vi "RT Driver VI.vi"(7 "Operation":T1, 11 "Device Reference in":T2 format="%.0x") -> (0 "Error Code":i32)   [LabVIEW 2015, in "Diagnostics Addon Engine.lvlib"]
uses:
  Diagnostics Addon Engine.lvlib
  <vilib>/NI Veristand/Custom Device API/Custom Device Item Ref.ctl
  <vilib>/NI Veristand/Custom Device API/Hardware Interface Driver VI Operation.ctl
  SubVIs/Inline Async API/Controls/Parameters Cluster.ctl
  SubVIs/Error Handling API/Controls/Error Handling Cluster.ctl
  SubVIs/VS Data Channels.ctl
  SubVIs/Inline Async API/Controls/Write To VS Engine.ctl
  <vilib>/NI Veristand/Custom Device API/Data Reference.ctl
  SubVIs/Inline Async API/Controls/Read From VS Engine.ctl
  <vilib>/NI Veristand/Custom Device API/Block Data Reference.ctl
  SubVIs/Inline Async API/Controls/ReadWrite Data.ctl
  SubVIs/Compiled.Settings
  SubVIs/Section Properties.ctl
  Shared/CAN Configuration.ctl
  Shared/CAN Interface.ctl
  Shared/Diagnostic Protocols.ctl
  Shared/Transport Protocols.ctl
  Shared/Security.ctl
  Shared/FPGA Bitfile Settings.ctl
  Shared/Frame Parameters.ctl
  Shared/Signal Parameters.ctl
  Shared/DPID Parameters.ctl
  Shared/DPID Periodic Rate.ctl
  <vilib>/Automotive Diagnostic Command Set/Diagnostic Protocols.llb/DTC Descriptor.ctl
  Shared/Compiled.Refs.ctl
  SubVIs/Inline Async API/Initialize Read From VS Engine.vi
  <vilib>/NI Veristand/Custom Device API/NI VeriStand - Set Channel Value by Data Reference.vi
  <vilib>/NI Veristand/Custom Device API/NI VeriStand - Get Channel Value by Data Reference.vi
  <vilib>/NI Veristand/Custom Device API/NI VeriStand - Get Channel Values by Block Data Reference.vi
  SubVIs/Error Handling API/Print/Display and Log Custom Device Error.vi
  Shared/GUID Lookup.vi
  <vilib>/NI Veristand/Custom Device API/Get Item Property (Variant).vi
  SubVIs/Read and Load Bitfile.vi
  SubVIs/Inline Async API/Initialize ReadWrite Data.vi
  SubVIs/Inline Async API/Initialize Write Data to VS Engine.vi
  <vilib>/NI Veristand/Custom Device API/Global Data Refs.vi
  SubVIs/Inline Async API/Inline Async API.lvlib
  SubVIs/Error Handling API/Error Handling API.lvlib
  <vilib>/NI Veristand/Custom Device API/Custom Device API.lvlib
  <vilib>/NI Veristand/Custom Device Tools/Custom Device Utility Library/Custom Device Utility Library.lvlib
  Shared/Diagnostics Addon Shared.lvlib
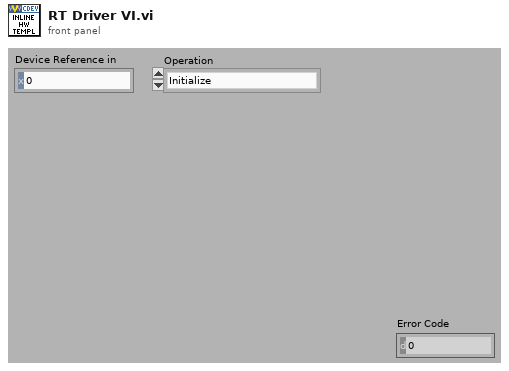
[diagram p1: front panel]
types:
  T1 = typedef "Custom Device API.lvlib/Hardware Interface Driver VI Operation.ctl" = enum16{"Initialize", "Start", "Read Data from HW", "Write Data to HW", "Close"}
  T2 = typedef "Custom Device API.lvlib/Custom Device Item Ref.ctl" = u64
  T3 = typedef "Diagnostics Addon Engine.lvlib/Error Handling API.lvlib/Error Handling Cluster.ctl" = cluster{"Error Process Q":refnum<queue>, "Process Qs":refnum<queue>[]}
  T4 = typedef "Diagnostics Addon Engine.lvlib/VS Data Channels.ctl" = cluster{"ToVS.PIDs":T5, "ToVS.DIDs":T5, "ToVS.DTCs":T5, "ToVS.DTCCount":T5, "ToVS.Success":T5, "FromVS.CPIDs":T7, "Cmds":T9}
  T5 = typedef "Diagnostics Addon Engine.lvlib/Inline Async API.lvlib/Write To VS Engine.ctl" = cluster{"Name":string, "Write to VS Engine FIFO":refnum<k33>, "Pairs":cluster{"Refs":T6[], "Values":dbl[]}}
  T6 = typedef "Custom Device API.lvlib/Data Reference.ctl" = i32
  T7 = typedef "Diagnostics Addon Engine.lvlib/Inline Async API.lvlib/Read From VS Engine.ctl" = cluster{"Name":string, "Read from VS Engine FIFO":refnum<k33>, "Pairs":cluster{"Refs":T8[], "Values":dbl[]}}
  T8 = typedef "Custom Device API.lvlib/Block Data Reference.ctl" = cluster{"Data Reference":T6, "Offset":u64, "Length":u64}
  T9 = typedef "Diagnostics Addon Engine.lvlib/Inline Async API.lvlib/ReadWrite Data.ctl" = cluster{"Name":string, "Write to VS Engine FIFO":refnum<k33>, "Read from VS Engine FIFO":refnum<k33>, "Pairs":cluster{"Chan Refs":T6[], "Prev. Values":dbl[]}}
  T10 = cluster{"Device Error":errorcluster, "VI Refs":refnum<vi>[], "Error Handling Cluster":T3, "ChanRefs":T4, "FPGA Session":u32}
  T11 = typedef "Diagnostics Addon Shared.lvlib/Compiled.Settings" = cluster{"Properties":T12, "Refs":T24}
  T12 = typedef "Diagnostics Addon Engine.lvlib/Section Properties.ctl" = cluster{"Name":string, "CAN":T13, "FPGA Settings":T18, "PIDs":T19[], "PID Lookup":variant, "CPIDs":T19[], "CPID Lookup":variant, "DIDs":T19[], "DID Lookup":variant, "DPIDs":T21[], "DPID Lookup":variant, "DTC descriptor":T23}
  T13 = typedef "Diagnostics Addon Shared.lvlib/CAN Configuration.ctl" = cluster{"Database File":path, "CAN Interface":T14, "Baud Rate":u32, "Diagnostic Protocol":T15, "Transport Protocol":T16, "Transmit ID":u32, "Receive ID":u32, "Transmit Extension":u8, "Receive Extension":u8, "Receive UUDT ID":u32, "Enable Stream":bool, "VW TP Channel ID":u32, "Security":T17}
  T14 = typedef "Diagnostics Addon Shared.lvlib/CAN Interface.ctl" = enum16{"CAN0", "CAN1", "CAN2", "CAN3", "CAN4", "CAN5", "CAN6", "CAN7", "CAN8", "CAN9", "CAN10", "CAN11", "CAN12", "CAN13", "CAN14", "CAN15", "CAN16", "CAN17", "CAN18", "CAN19", "CAN20", "CAN21", "CAN22", "CAN23", "CAN24", "CAN25", "CAN26", "CAN27", "CAN28", "CAN29", "CAN30", "CAN31", "CAN32", "CAN33", "CAN34", "CAN35", "CAN36", "CAN37", "CAN38", "CAN39", "CAN40", "CAN41", "CAN42", "CAN43", "CAN44", "CAN45", "CAN46", "CAN47", "CAN48", "CAN49", "CAN50", "CAN51", "CAN52", "CAN53", "CAN54", "CAN55", "CAN56", "CAN57", "CAN58", "CAN59", "CAN60", "CAN61", "CAN62", "CAN63", "CAN 256 (Virtual)", "CAN 257 (Virtual)"}
  T15 = typedef "Diagnostics Addon Shared.lvlib/Diagnostic Protocols.ctl" = enum16{"GMLAN", "KWP-2000", "UDS"}
  T16 = typedef "Diagnostics Addon Shared.lvlib/Transport Protocols.ctl" = enum16{"ISO TP - Normal Mode", "ISO TP - Mixed Mode", "VW TP 2.0", "Diagnostics on IP"}
  T17 = typedef "Diagnostics Addon Shared.lvlib/Security.ctl" = cluster{"DLL Path":path, "Security Level":u8}
  T18 = typedef "Diagnostics Addon Shared.lvlib/FPGA Bitfile Settings.ctl" = cluster{"RT Bitfile Path":path, "RIO Device":u16, "Enable":bool}
  T19 = typedef "Diagnostics Addon Shared.lvlib/Frame Parameters.ctl" = cluster{"Name":string, "Description":string, "ID":u16, "Signals":T20[]}
  T20 = typedef "Diagnostics Addon Shared.lvlib/Signal Parameters.ctl" = cluster{"Start Bit":u8, "Length":u8, "Scaling Factor":dbl, "Scaling Offset":dbl, "Minimum":dbl, "Maximum":dbl, "Data Type":u32, "Byte Order":u32, "Default Value":dbl, "Name":string, "Units":string, "Description":string}
  T21 = typedef "Diagnostics Addon Shared.lvlib/DPID Parameters.ctl" = cluster{"DPID ID":u8, "Speed":T22, "PIDs":u16[]}
  T22 = typedef "Diagnostics Addon Shared.lvlib/DPID Periodic Rate.ctl" = enum16{"Slow", "Medium", "Fast"}
  T23 = typedef "Diagnostics Addon Shared.lvlib/DTC Descriptor.ctl" = cluster{"DTC Byte Length":i32, "Status Byte Length":i32, "Add Data Byte Length":i32, "Byte Order":enum16{"Motorola", "Intel"}}
  T24 = typedef "Diagnostics Addon Shared.lvlib/Compiled.Refs.ctl" = cluster{"PIDs":T6[], "CPIDs":cluster{"Refs":T8[], "Values":dbl[]}, "DIDs":T6[], "Number of DTCs":T6, "DTCs":T6[], "Success":T6, "Command Chanels":T6[]}
  T25 = typedef "Diagnostics Addon Engine.lvlib/Inline Async API.lvlib/Parameters Cluster.ctl" = cluster{"Parameter Name":string, "Initial Settings":variant}
  T26 = typedef "Diagnostics Addon Engine.lvlib/Main Configuration.ctl" = cluster{"Properties":T12, "ChanRefs":T4}
  T27 = cluster{"Chan Refs":T6[], "Previous Chan Values":dbl[]}
  T28 = cluster{"Block Data Refs":T8[], "Previous Chan Values":dbl[]}
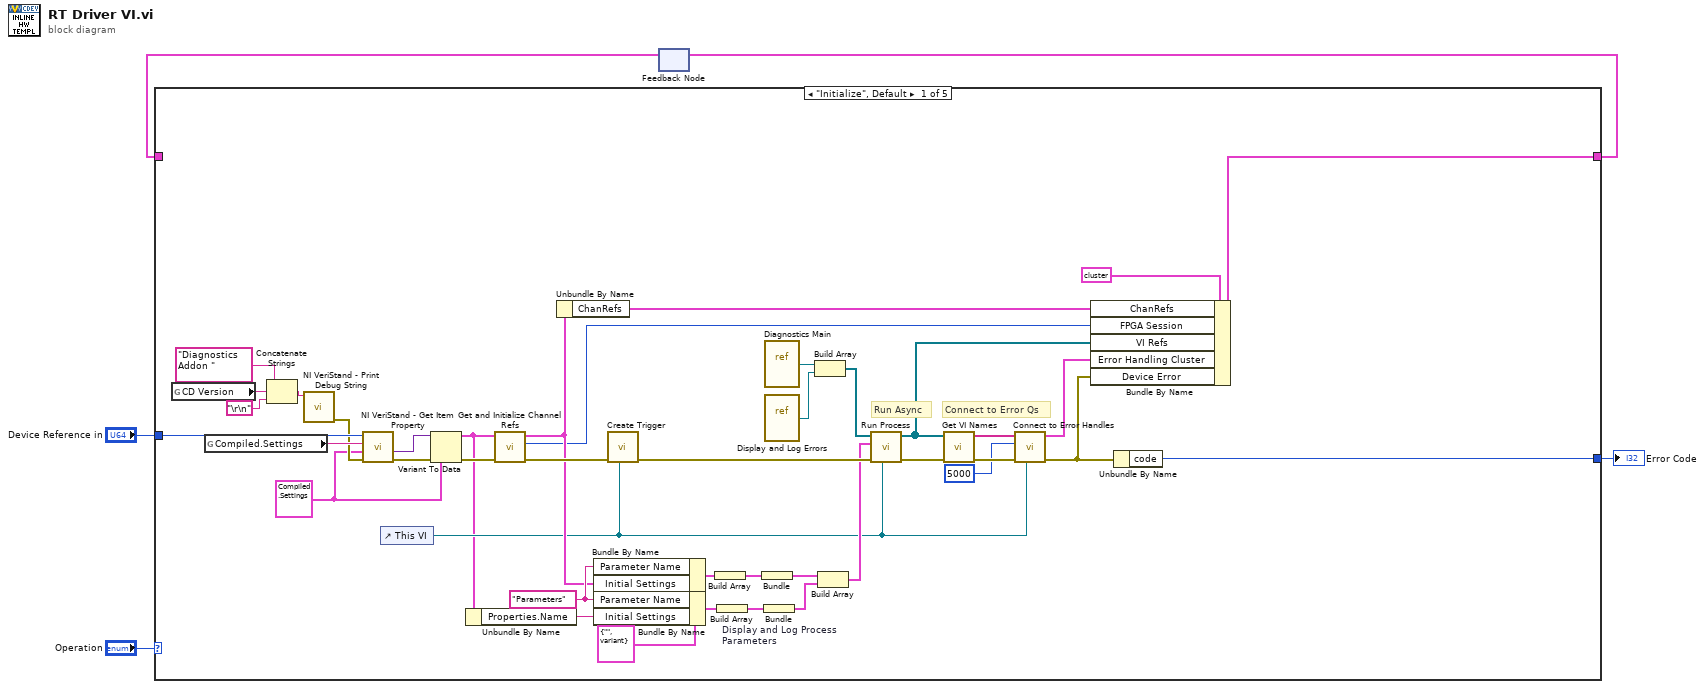
[diagram p0: block diagram]
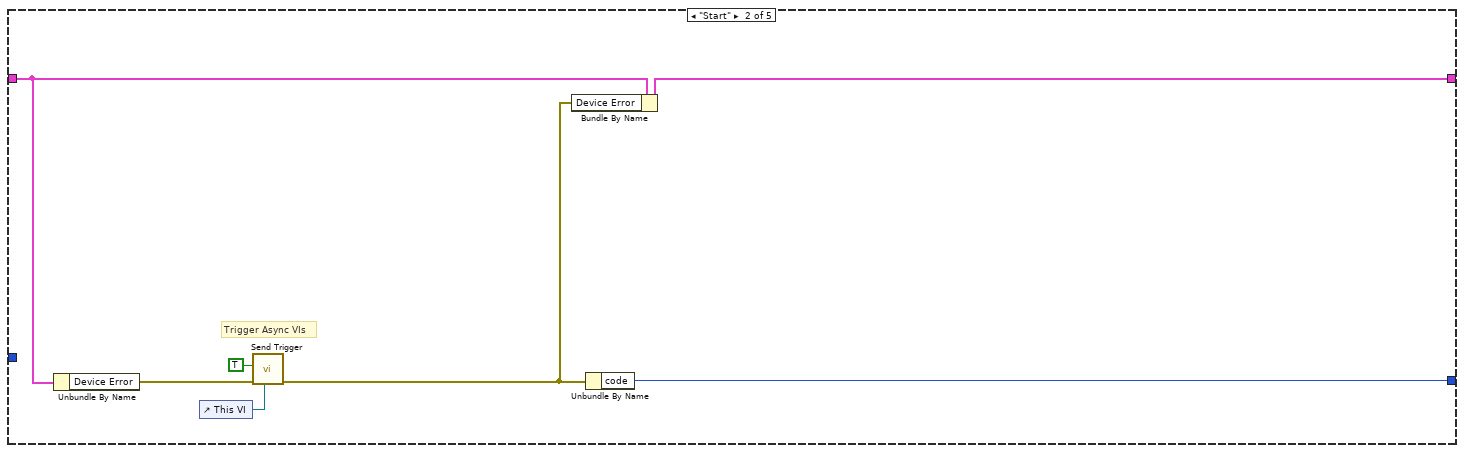
[diagram p2: hidden frame]
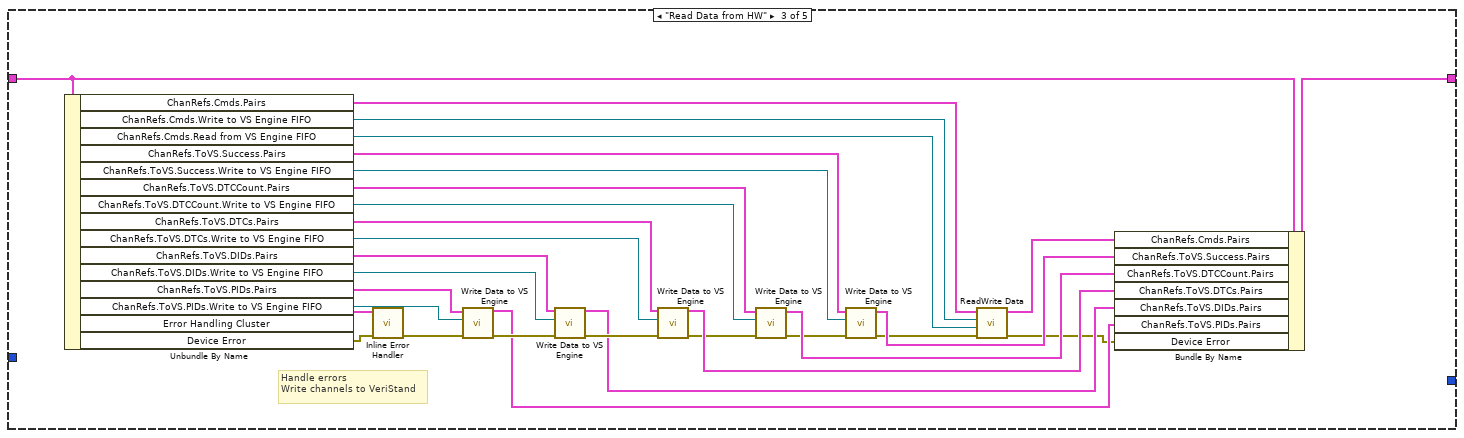
[diagram p3: hidden frame]
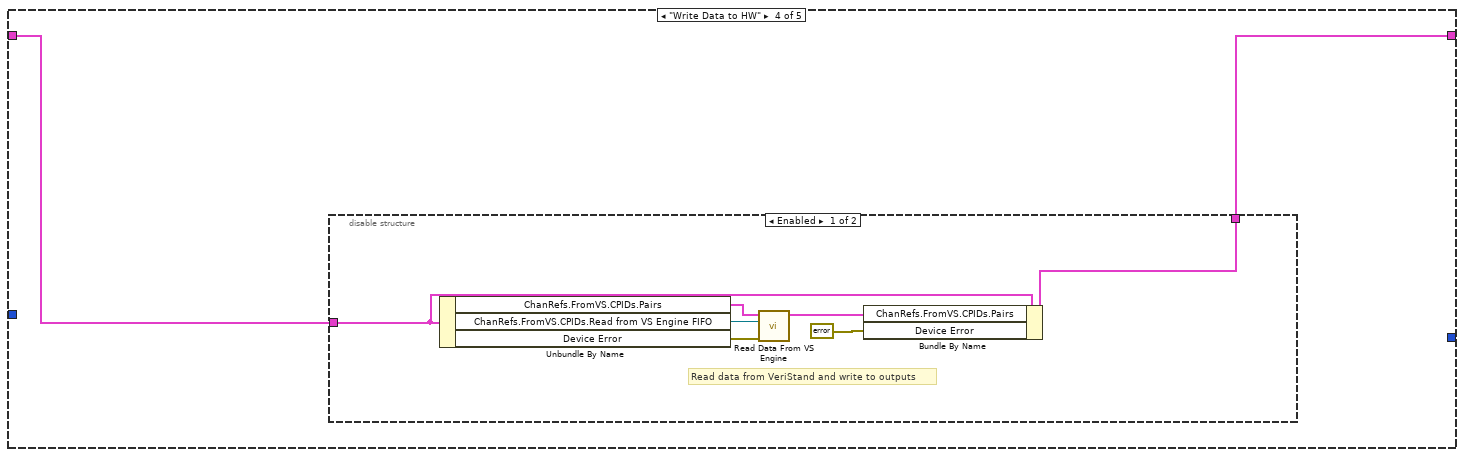
[diagram p4: hidden frame]
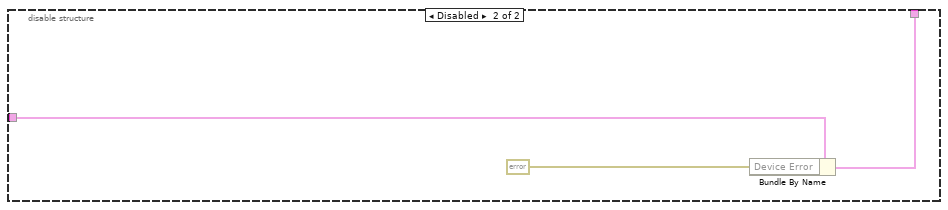
[diagram p5: hidden frame]
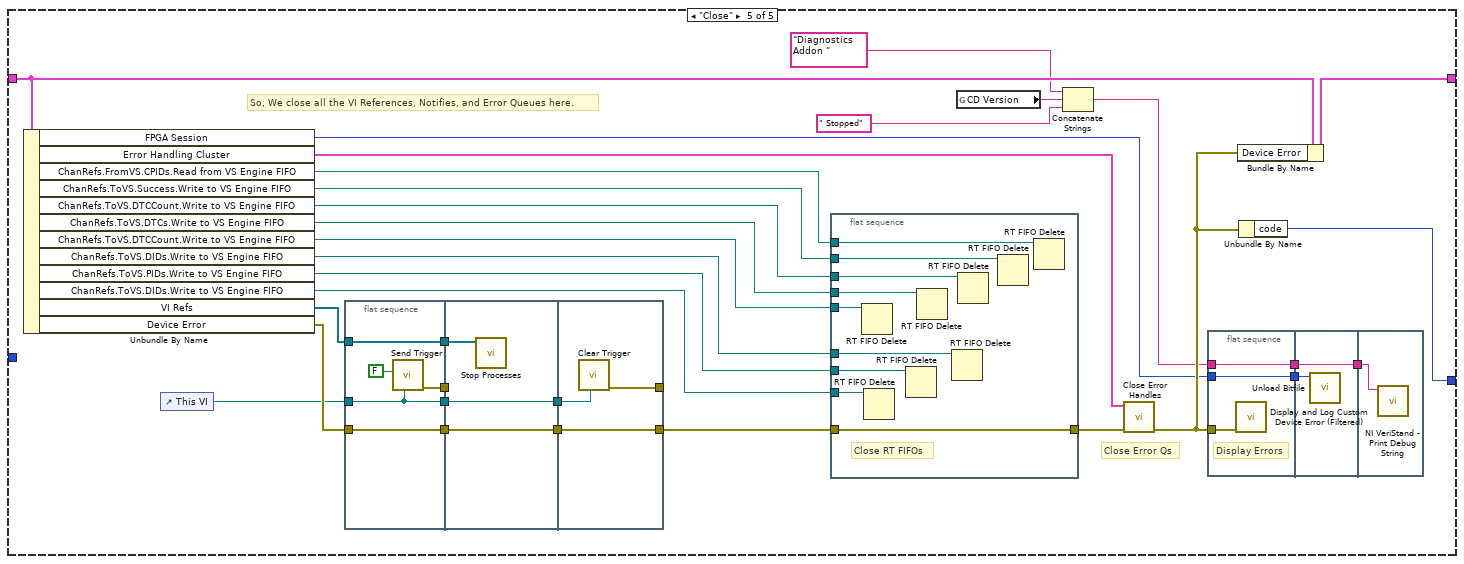
[diagram p6: hidden frame]
diagram:
  n1 = feedback #1() -> (w3:T10)  [unwired: 1 out]
  n2 = case shown="\"Initialize\", Default" "Operation" {
    tunnel: [w36 w51 w82 w84 w126] -> w1
    tunnel: w3 -> [_ w52 w83 w85 w125]
    tunnel: "Device Reference in" -> [w14 _ _ _ _]
    tunnel: [w46 w53 _ _ w127] -> w2
    frame "Initialize", Default {
      w10 = T11 {"Properties"={"Name"="", "CAN"={"Database File"=path "", "CAN Interface"=enum."CAN1", "Baud Rate"=0, "Diagnostic Protocol"=enum."GMLAN", "Transport Protocol"=enum."ISO TP - Normal Mode", "Transmit ID"=0, "Receive ID"=0, "Transmit Extension"=2, "Receive Extension"=1, "Receive UUDT ID"=0, "Enable Stream"=TRUE, "VW TP Channel ID"=0, "Security"={"DLL Path"=path "", "Security Level"=0}}, "FPGA Settings"={"RT Bitfile Path"=path "", "RIO Device"=0, "Enable"=FALSE}, "PIDs"=[], "PID Lookup"=variant(enum16{"GMLAN", "KWP-2000", "UDS"} enum."GMLAN"), "CPIDs"=[], "CPID Lookup"=variant(u32 0), "DIDs"=[], "DID Lookup"=variant(u8 0), "DPIDs"=[], "DPID Lookup"=variant(u32 0), "DTC descriptor"={"DTC Byte Length"=2, "Status Byte Length"=1, "Add Data Byte Length"=1, "Byte Order"=enum."Motorola"}}, "Refs"={"PIDs"=[], "CPIDs"={"Refs"=[], "Values"=[]}, "DIDs"=[], "Number of DTCs"=0, "DTCs"=[], "Success"=0, "Command Chanels"=[]}} ("VS References")
      w29 = "Parameters" ("Parameter Name")
      w26 = T25 {"Parameter Name"="", "Initial Settings"=variant} ("Parameters")
      # "Connect to Error Qs"
      # "Run Async"
      n3 = global read "GUID Lookup.vi" "CD Version"() -> (w21:string)
      n4 = global read "GUID Lookup.vi" "Compiled.Settings"() -> (w15:string)
      n5 = Concatenate Strings("Diagnostics Addon " ("string"), w21, "\r\n") -> (w19:string)
      n6 = call <vilib>:"NI VeriStand - Print Debug String.vi"("Message"=w19) -> ("error out"=w13:errorcluster)  [unwired: 10 in]
      n7 = call-poly <vilib>:"NI VeriStand - Get Item Property.vi"("error in (no error)"=w13, "Default Value"=w10, "Property Name"=w15, "Item Ref in"=w14) -> ("error out"=w12:errorcluster, "Value"=w11:variant)  [unwired: 4 in, 2 out]
      n8 = control-ref of="This VI"() -> (w22:refnum<vi>)
      n9 = Variant To Data(error in=w12, type=w10, Variant=w11) -> (data=w8:T11, error out=w9:errorcluster)
      n10 = Unbundle By Name(w8) -> ("Properties.Name"=w7:string)
      n11 = call "Get and Initialize Channel Refs.vi"("error in (no error)"=w9, "VS References"=w8) -> ("error out"=w34:errorcluster, "FPGA Session"=w6:u32, "VS Main Configuration"=w24:T26)  [unwired: 7 in]
      n12 = Unbundle By Name(w24) -> ("ChanRefs"=w23:T4)
      n13 = Bundle By Name(cluster=w26, "Parameter Name"=w29, "Initial Settings"=w24) -> (w27:T25)
      n14 = Bundle By Name(cluster=w26, "Parameter Name"=w29, "Initial Settings"=w7) -> (w33:T25)
      n15 = call "Create Trigger.vi"("This VI"=w22, "error in (no error)"=w34) -> ("error out"=w41:errorcluster)  [unwired: 9 in]
      n16 = Build Array(w27) -> (w28:T25[])
      n17 = Build Array(w33) -> (w32:T25[])
      n18 = Bundle ("Display and Log Process Parameters")(w28) -> (w25:cluster{T25[]})  [unwired: 1 in]
      n19 = Bundle "Display and Log Process Parameters"(w32) -> (w31:cluster{T25[]})  [unwired: 1 in]
      n20 = vi-ref "Diagnostics Main.vi"() -> (w35:refnum<vi>)
      n21 = vi-ref "Display and Log Errors.vi"() -> (w45:refnum<vi>)
      n22 = Build Array(w35, w45) -> (w42:refnum<vi>[])
      n23 = Build Array(w25, w31) -> (w30:cluster{T25[]}[])
      n24 = call "Run Process.vi"("Parent VI"=w22, "error in (no error)"=w41, "Initial Parameters"=w30, "VI Ref In"=w42) -> ("error out"=w40:errorcluster, "VI Ref In"=w39:refnum<vi>[])  [unwired: 6 in]
      n25 = call "Get VI Names.vi"("error in"=w40, "VI References"=w39) -> ("error out"=w44:errorcluster, "Clone Names"=w38:string[])  [unwired: 8 in]
      n26 = call "Connect to Error Handles.vi"("Parent"=w22, "error in"=w44, "Timeout (ms)"=u16 5000, "Process Names"=w38) -> ("error out"=w20:errorcluster, "Error Handling Cluster"=w43:T3)  [unwired: 6 in]
      n27 = Bundle By Name(cluster=T10 {"Device Error"={"status"=FALSE, "code"=0, "source"=""}, "VI Refs"=[], "Error Handling Cluster"={"Error Process Q"=refnum, "Process Qs"=[]}, "ChanRefs"={"ToVS.PIDs"={"Name"="", "Write to VS Engine FIFO"=refnum, "Pairs"={"Refs"=[], "Values"=[]}}, "ToVS.DIDs"={"Name"="", "Write to VS Engine FIFO"=refnum, "Pairs"={"Refs"=[], "Values"=[]}}, "ToVS.DTCs"={"Name"="", "Write to VS Engine FIFO"=refnum, "Pairs"={"Refs"=[], "Values"=[]}}, "ToVS.DTCCount"={"Name"="", "Write to VS Engine FIFO"=refnum, "Pairs"={"Refs"=[], "Values"=[]}}, "ToVS.Success"={"Name"="", "Write to VS Engine FIFO"=refnum, "Pairs"={"Refs"=[], "Values"=[]}}, "FromVS.CPIDs"={"Name"="", "Read from VS Engine FIFO"=refnum, "Pairs"={"Refs"=[], "Values"=[]}}, "Cmds"={"Name"="", "Write to VS Engine FIFO"=refnum, "Read from VS Engine FIFO"=refnum, "Pairs"={"Chan Refs"=[], "Prev. Values"=[]}}}, "FPGA Session"=0}, "ChanRefs"=w23, "FPGA Session"=w6, "VI Refs"=w39, "Error Handling Cluster"=w43, "Device Error"=w20) -> (w36:T10)
      n28 = Unbundle By Name(w20) -> ("code"=w46:i32)
    }
    frame "Start" {
      # "Trigger Async VIs"
      n29 = Unbundle By Name(w52) -> ("Device Error"=w50:errorcluster)
      n30 = control-ref of="This VI"() -> (w47:refnum<vi>)
      n31 = call "Send Trigger.vi"("Parent VI"=w47, "error in (no error)"=w50, "notification"=TRUE) -> ("error out"=w49:errorcluster)  [unwired: 8 in]
      n32 = Bundle By Name(cluster=w52, "Device Error"=w49) -> (w51:T10)
      n33 = Unbundle By Name(w49) -> ("code"=w53:i32)
    }
    frame "Read Data from HW" {
      # "Handle errors\nWrite channels to VeriStand"
      n34 = Unbundle By Name(w83) -> ("ChanRefs.Cmds.Pairs"=w59:cluster{"Chan Refs":T6[], "Prev. Values":dbl[]}, "ChanRefs.Cmds.Write to VS Engine FIFO"=w57:refnum<k33>, "ChanRefs.Cmds.Read from VS Engine FIFO"=w56:refnum<k33>, "ChanRefs.ToVS.Success.Pairs"=w62:cluster{"Refs":T6[], "Values":dbl[]}, "ChanRefs.ToVS.Success.Write to VS Engine FIFO"=w61:refnum<k33>, "ChanRefs.ToVS.DTCCount.Pairs"=w65:cluster{"Refs":T6[], "Values":dbl[]}, "ChanRefs.ToVS.DTCCount.Write to VS Engine FIFO"=w66:refnum<k33>, "ChanRefs.ToVS.DTCs.Pairs"=w73:cluster{"Refs":T6[], "Values":dbl[]}, "ChanRefs.ToVS.DTCs.Write to VS Engine FIFO"=w72:refnum<k33>, "ChanRefs.ToVS.DIDs.Pairs"=w75:cluster{"Refs":T6[], "Values":dbl[]}, "ChanRefs.ToVS.DIDs.Write to VS Engine FIFO"=w74:refnum<k33>, "ChanRefs.ToVS.PIDs.Pairs"=w77:cluster{"Refs":T6[], "Values":dbl[]}, "ChanRefs.ToVS.PIDs.Write to VS Engine FIFO"=w81:refnum<k33>, "Error Handling Cluster"=w78:T3, "Device Error"=w80:errorcluster)
      n35 = call "Inline Error Handler.vi"("error in"=w80, "Error Handling Cluster"=w78) -> ("error out"=w79:errorcluster)  [unwired: 9 in]
      n36 = call "Write Data to VS Engine.vi"("error in"=w79, "Write to VS Engine FIFO"=w81, "Channel Pairs"=w77) -> ("error out"=w76:errorcluster, "Channel Pairs Out"=w70:T27)  [unwired: 6 in, 1 out]
      n37 = call "Write Data to VS Engine.vi"("error in"=w76, "Write to VS Engine FIFO"=w74, "Channel Pairs"=w75) -> ("error out"=w71:errorcluster, "Channel Pairs Out"=w69:T27)  [unwired: 6 in, 1 out]
      n38 = call "Write Data to VS Engine.vi"("error in"=w71, "Write to VS Engine FIFO"=w72, "Channel Pairs"=w73) -> ("error out"=w67:errorcluster, "Channel Pairs Out"=w68:T27)  [unwired: 6 in, 1 out]
      n39 = call "Write Data to VS Engine.vi"("error in"=w67, "Write to VS Engine FIFO"=w66, "Channel Pairs"=w65) -> ("error out"=w63:errorcluster, "Channel Pairs Out"=w64:T27)  [unwired: 6 in, 1 out]
      n40 = call "Write Data to VS Engine.vi"("error in"=w63, "Write to VS Engine FIFO"=w61, "Channel Pairs"=w62) -> ("error out"=w55:errorcluster, "Channel Pairs Out"=w60:T27)  [unwired: 6 in, 1 out]
      n41 = call "ReadWrite Data.vi"("error in"=w55, "Read from VS Engine FIFO"=w56, "Write to VS Engine FIFO"=w57, "Channel Pairs"=w59) -> ("error out"=w54:errorcluster, "Channel Pairs Out"=w58:T27)  [unwired: 5 in, 1 out]
      n42 = Bundle By Name(cluster=w83, "ChanRefs.Cmds.Pairs"=w58, "ChanRefs.ToVS.Success.Pairs"=w60, "ChanRefs.ToVS.DTCCount.Pairs"=w64, "ChanRefs.ToVS.DTCs.Pairs"=w68, "ChanRefs.ToVS.DIDs.Pairs"=w69, "ChanRefs.ToVS.PIDs.Pairs"=w70, "Device Error"=w54) -> (w82:T10)
    }
    frame "Write Data to HW" {
      n43 = disable-structure shown="Enabled" {
        disable-tunnel: w85 -> [w92 w95]
        disable-tunnel: [w91 w94] -> w84
        frame Enabled {
          # "Read data from VeriStand and write to outputs"
          n44 = Unbundle By Name(w92) -> ("ChanRefs.FromVS.CPIDs.Pairs"=w88:cluster{"Refs":T8[], "Values":dbl[]}, "ChanRefs.FromVS.CPIDs.Read from VS Engine FIFO"=w89:refnum<k33>, "Device Error"=w90:errorcluster)
          n45 = call "Read Data From VS Engine.vi"("error in"=w90, "Read from VS Engine FIFO"=w89, "Channel Pairs"=w88) -> ("Channel Pairs"=w87:T28)  [unwired: 6 in, 2 out]
          n46 = Bundle By Name(cluster=w92, "ChanRefs.FromVS.CPIDs.Pairs"=w87, "Device Error"=errorcluster {"status"=FALSE, "code"=0, "source"=""}) -> (w91:T10)
        }
        frame Disabled {
          n47 = Bundle By Name(cluster=w95, "Device Error"=errorcluster {"status"=FALSE, "code"=0, "source"=""}) -> (w94:T10)
        }
      }
    }
    frame "Close" {
      # "Close Error Qs"
      # "So, We close all the VI References, Notifies, and Error Queues here."
      n48 = Unbundle By Name(w125) -> ("FPGA Session"=w103:u32, "Error Handling Cluster"=w120:T3, "ChanRefs.FromVS.CPIDs.Read from VS Engine FIFO"=w104:refnum<k33>, "ChanRefs.ToVS.Success.Write to VS Engine FIFO"=w105:refnum<k33>, "ChanRefs.ToVS.DTCCount.Write to VS Engine FIFO"=w106:refnum<k33>, "ChanRefs.ToVS.DTCs.Write to VS Engine FIFO"=w107:refnum<k33>, "ChanRefs.ToVS.DTCCount.Write to VS Engine FIFO"=w108:refnum<k33>, "ChanRefs.ToVS.DIDs.Write to VS Engine FIFO"=w124:refnum<k33>, "ChanRefs.ToVS.PIDs.Write to VS Engine FIFO"=w123:refnum<k33>, "ChanRefs.ToVS.DIDs.Write to VS Engine FIFO"=w109:refnum<k33>, "VI Refs"=w113:refnum<vi>[], "Device Error"=w112:errorcluster)
      n49 = control-ref of="This VI"() -> (w98:refnum<vi>)
      n50 = flat-sequence {
        tunnel: w112 -> [w135]
        tunnel: w98 -> [w137]
        tunnel: [w138] -> w119
        tunnel: w113 -> [w138]
        tunnel: [w137] -> w118
        tunnel: [w136] -> w117
        tunnel: [w135] -> w116
        tunnel: w119 -> [w141]
        tunnel: [w140] -> w115
        tunnel: w118 -> [w140]
        tunnel: w117 -> [_]
        tunnel: [w139] -> w114
        tunnel: w116 -> [w139]
        tunnel: [w142] -> w111
        tunnel: w115 -> [w144]
        tunnel: [w143] -> _
        tunnel: w114 -> [w142]
        frame #0 {
          n51 = call "Send Trigger.vi"("Parent VI"=w137, "notification"=FALSE) -> ("error out"=w136:errorcluster)  [unwired: 9 in]
        }
        frame #1 {
          n52 = call "Stop Processes.vi"("VI Refs"=w141) -> ()  [unwired: 11 in]
        }
        frame #2 {
          n53 = call "Clear Trigger.vi"("Parent VI"=w144) -> ("error out"=w143:errorcluster)  [unwired: 10 in]
        }
      }
      n54 = flat-sequence {
        tunnel: [w153] -> w122
        tunnel: w111 -> [w153]
        tunnel: w124 -> [w151]
        tunnel: w123 -> [w152]
        tunnel: w109 -> [w150]
        tunnel: w108 -> [w149]
        tunnel: w107 -> [w148]
        tunnel: w106 -> [w147]
        tunnel: w105 -> [w146]
        tunnel: w104 -> [w145]
        frame #0 {
          # "Close RT FIFOs"
          n55 = RT FIFO Delete(0:w149) -> ()  [unwired: 2 in, 1 out]
          n56 = RT FIFO Delete(0:w150) -> ()  [unwired: 2 in, 1 out]
          n57 = RT FIFO Delete(0:w152) -> ()  [unwired: 2 in, 1 out]
          n58 = RT FIFO Delete(0:w148) -> ()  [unwired: 2 in, 1 out]
          n59 = RT FIFO Delete(0:w151) -> ()  [unwired: 2 in, 1 out]
          n60 = RT FIFO Delete(0:w147) -> ()  [unwired: 2 in, 1 out]
          n61 = RT FIFO Delete(0:w146) -> ()  [unwired: 2 in, 1 out]
          n62 = RT FIFO Delete(0:w145) -> ()  [unwired: 2 in, 1 out]
        }
      }
      n63 = global read "GUID Lookup.vi" "CD Version"() -> (w97:string)
      n64 = Concatenate Strings("Diagnostics Addon " ("string"), w97, " Stopped" ("string")) -> (w99:string)
      n65 = call "Close Error Handles.vi"("error in"=w122, "Error Handling Cluster"=w120) -> ("error out"=w121:errorcluster)  [unwired: 9 in]
      n66 = flat-sequence {
        tunnel: w121 -> [w130]
        tunnel: w103 -> [w129]
        tunnel: [w129] -> w102
        tunnel: [w128] -> w100
        tunnel: w99 -> [w128]
        tunnel: w102 -> [w132]
        tunnel: [w131] -> w101
        tunnel: w100 -> [w131]
        tunnel: w101 -> [w133]
        frame #0 {
          # "Display Errors"
          n67 = call "Display and Log Custom Device Error (Filtered).vi"("error in (no error)"=w130) -> ()  [unwired: 11 in]
        }
        frame #1 {
          n68 = call "Unload Bitfile.vi"("Session"=w132) -> ()  [unwired: 11 in]
        }
        frame #2 {
          n69 = call <vilib>:"NI VeriStand - Print Debug String.vi"("Message"=w133) -> ()  [unwired: 10 in, 1 out]
        }
      }
      n70 = Bundle By Name(cluster=w125, "Device Error"=w121) -> (w126:T10)
      n71 = Unbundle By Name(w121) -> ("code"=w127:i32)
    }
  }
  "Error Code" <- w2
  n72 = feedback-in #1(w1) -> ()
